vi "RegisterPublisher.vi"(6 "1:M":bool, 7 "Topic Name":string, 8 "error in (no error)":errorcluster, 11 "Message Broker in":refnum<class "Message Broker.lvclass">) -> (0 "error out":errorcluster, 2 "Topic Actor Created?":bool, 3 "Message Broker out":refnum<class "Message Broker.lvclass">, 4 "Locked?":bool, 5 "Transport":refnum<class "Message Transport Queue.lvclass">)   [LabVIEW 2016, in "Stream Mediator.lvlib" / "Message Broker.lvclass"]
doc: "--\nCopyright © 2017 Composed SystemsI All rights reserved.\n\nAuthor: Jon McBee <jon.mcbee@composed.io>\n\nThis library is provided \"AS IS\" ,WITHOUT WARRANTIES OR\nCONDITIONS OF ANY KIND, either express or implied.\n\nComposed Systems -- composed.io\n\nStream 0.0.1.1\nJon McBee - Composed Systems\nCopyright (c) 2017, Composed Systems"
uses:
  <userlib>/Composed Systems/Stream/Mediator/Classes/Message Broker/Message Broker.lvclass
  <userlib>/Composed Systems/Stream/Mediator/Classes/Message Transport Queue/Message Transport Queue.lvclass
  <userlib>/Composed Systems/Stream/Mediator/Classes/Message Broker/Message Broker.lvclass/Message Broker.ctl
  <userlib>/Composed Systems/Stream/Mediator/Classes/Topic Actor Look Up Table/Topic Actor Look Up Table.lvclass
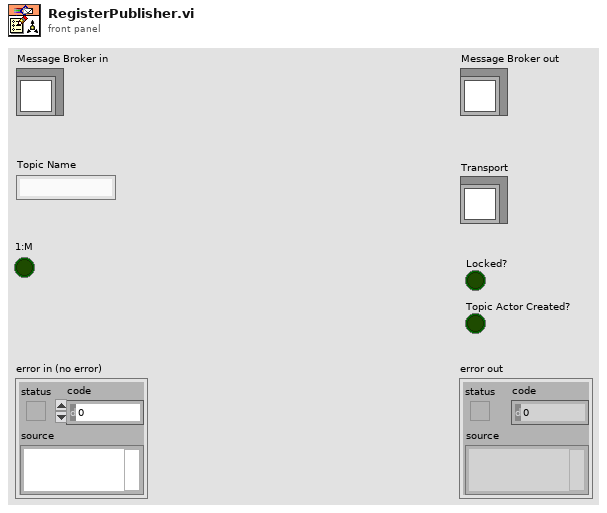
[diagram p1: front panel]
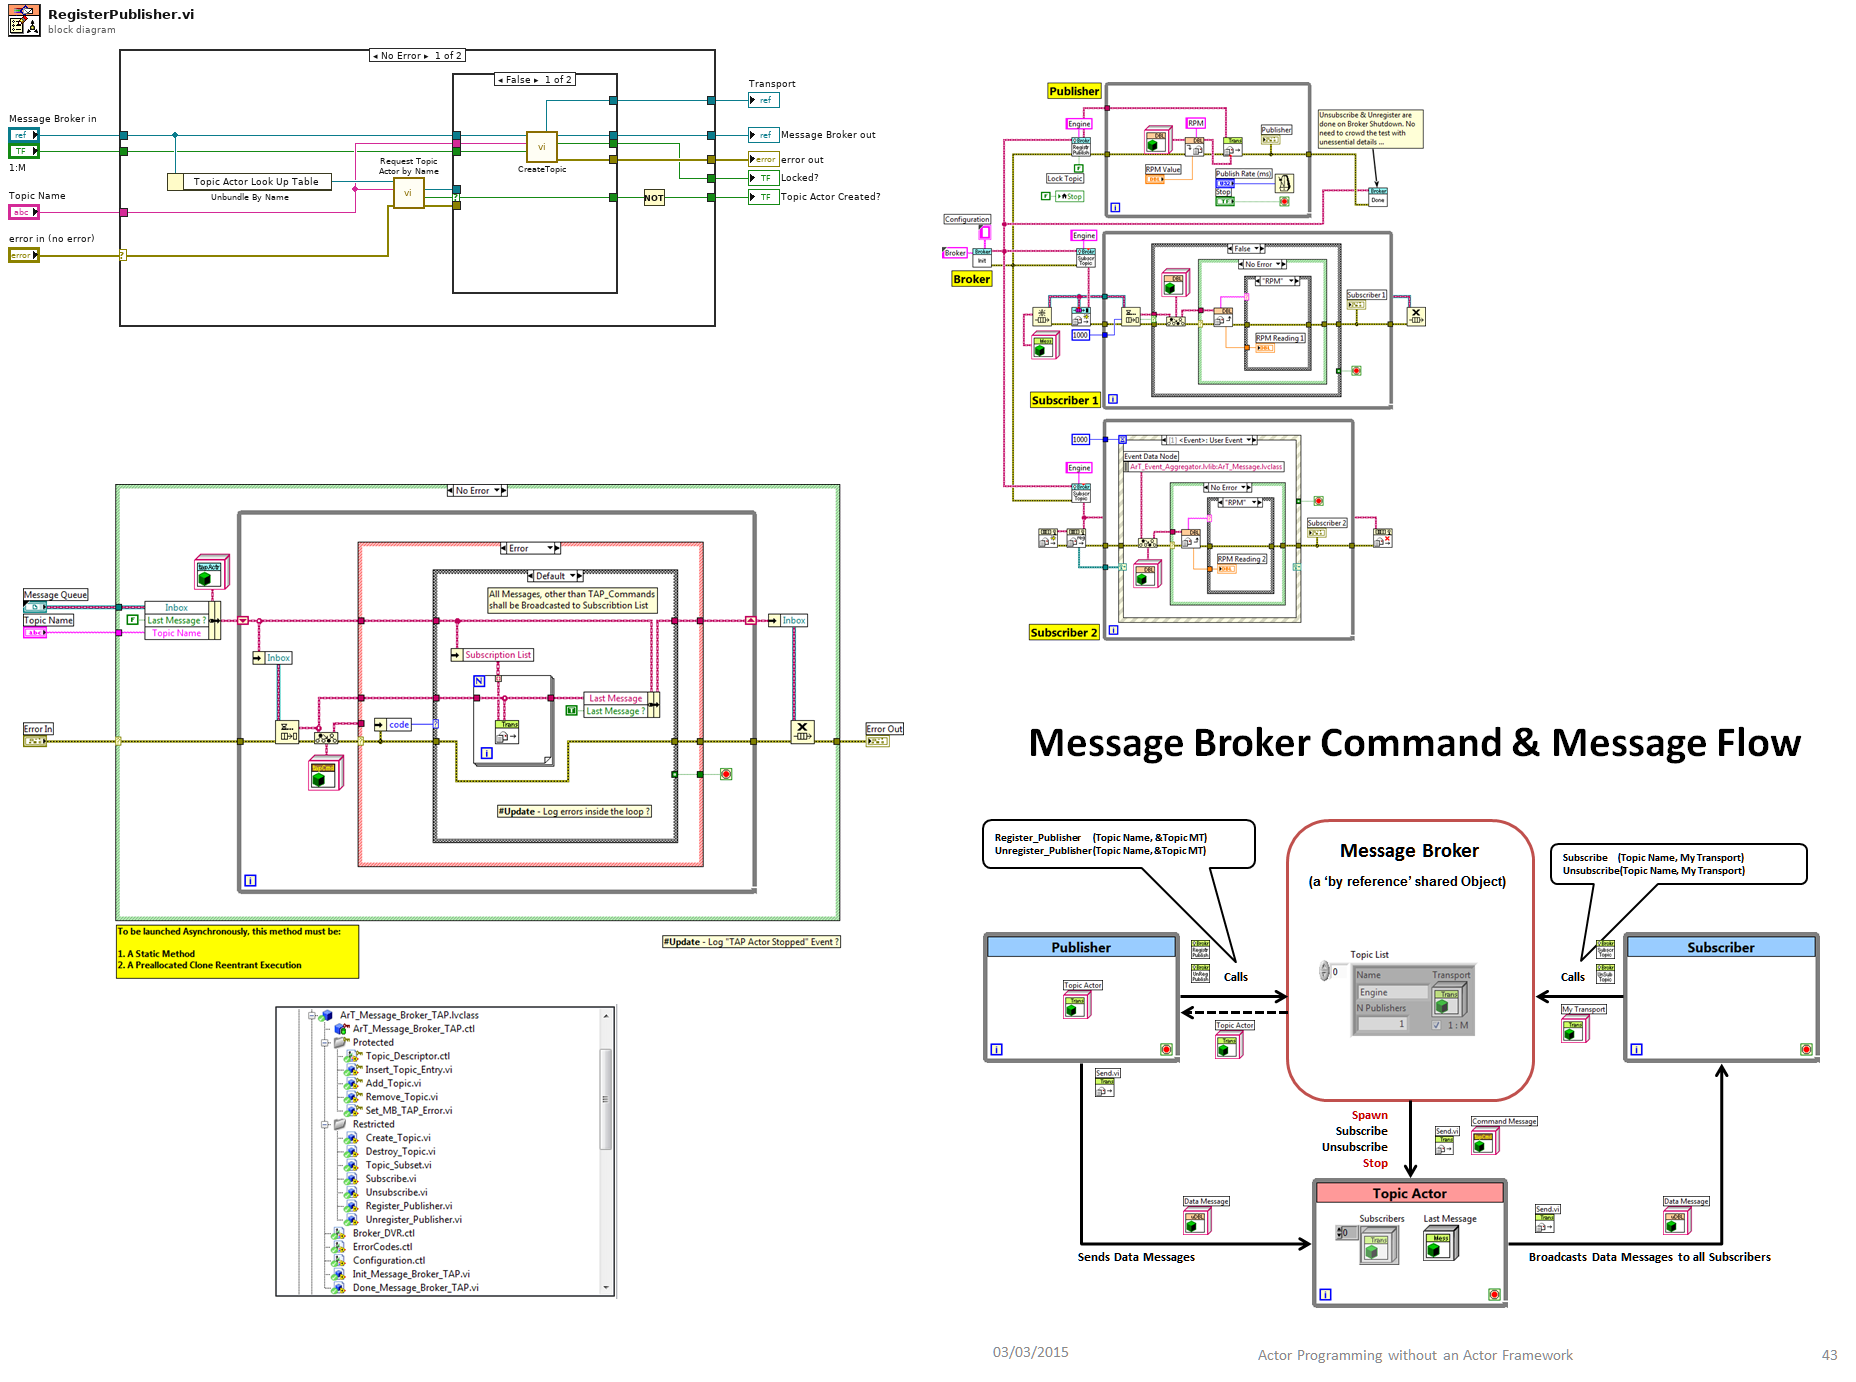
[diagram p0: block diagram]
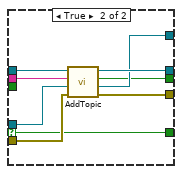
[diagram p2: hidden frame]
diagram:
  n1 = case shown="No Error" "error in (no error)" {
    selector: "error in (no error)" -> [w22 w42]
    tunnel: [w14 w42] -> w8
    tunnel: [w20 w41] -> w6
    tunnel: "Message Broker in" -> [w21 w41]
    tunnel: "Topic Name" -> [w18 _]
    tunnel: "1:M" -> [w17 _]
    tunnel: [w15 _] -> w3
    tunnel: [w12 _] -> w2
    tunnel: [w10 _] -> w1
    frame No Error {
      n2 = Unbundle By Name(w21) -> ("Topic Actor Look Up Table"=w23:refnum<class "Topic Actor Look Up Table.lvclass">)
      n3 = call <userlib>:"Request Topic Actor by Name.vi"("error in (no error)"=w22, "Topic Actor"=w18, "Topic Actor Look Up Table in"=w23) -> ("error out"=w16:errorcluster, "Found?"=w19:bool, "Topic Actor Descriptor"=w13:refnum<class "Topic Actor Descriptor.lvclass">)  [unwired: 5 in, 1 out]
      n4 = case shown="False" w19 {
        selector: w19 -> [w24 w32]
        tunnel: w21 -> [w31 w40]
        tunnel: [w30 w39] -> w20
        tunnel: w18 -> [w29 w38]
        tunnel: w17 -> [w28 _]
        tunnel: w16 -> [_ w36]
        tunnel: [w27 w34] -> w15
        tunnel: [w26 w35] -> w14
        tunnel: w13 -> [_ w37]
        tunnel: [w25 w33] -> w12
        tunnel: [w24 w32] -> w11
        frame False {
          n5 = call-dynamic "CreateTopic.vi"("1:M"=w28, "Topic Name"=w29, "Message Broker in"=w31) -> ("error out"=w26:errorcluster, "Locked?"=w25:bool, "Message Broker out"=w30:refnum<class "Message Broker.lvclass">, "Transport"=w27:refnum<class "Message Transport Queue.lvclass">)  [unwired: 5 in]
        }
        frame True {
          n6 = call <userlib>:"AddTopic.vi"("error in (no error)"=w36, "Topic Actor Descriptor"=w37, "Topic Name"=w38, "Message Broker in"=w40) -> ("error out"=w35:errorcluster, "Transport"=w34:refnum<class "Message Transport Queue.lvclass">, "Locked?"=w33:bool, "Message Broker out"=w39:refnum<class "Message Broker.lvclass">)  [unwired: 4 in]
        }
      }
      n7 = Not(x=w11) -> (.not. x?=w10:bool)
    }
    frame Error {
    }
  }
  "error out" <- w8
  "Message Broker out" <- w6
  "Transport" <- w3
  "Locked?" <- w2
  "Topic Actor Created?" <- w1
